vi "New Signal DVR.vi"(8 "error in (no error)":errorcluster, 11 "Signal in":refnum<class "Signal.lvclass">) -> (0 "error out":errorcluster, 3 "Signal DVR out":refnum<data-value>)   [LabVIEW 2015, in "MDSplus.lvlib" / "Signal.lvclass"]
uses:
  <vilib>/MDSplus/Classes/Data_Class/Compound_Class/Signal_Class/Signal.lvclass
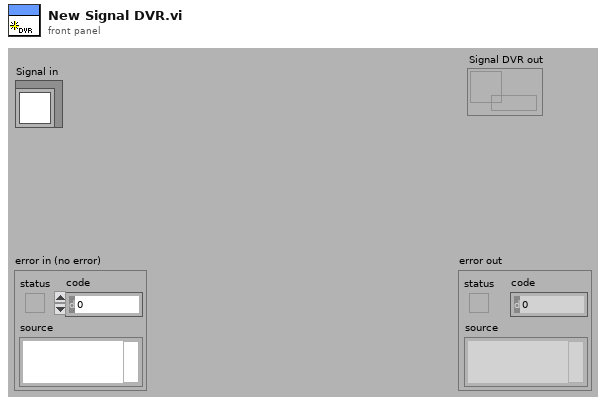
[diagram p1: front panel]
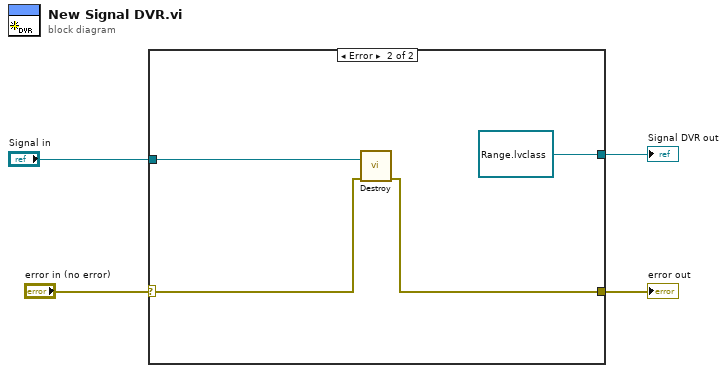
[diagram p0: block diagram]
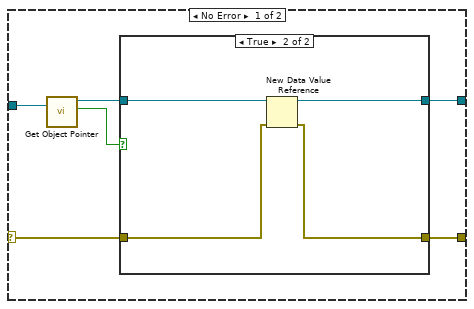
[diagram p2: hidden frame]
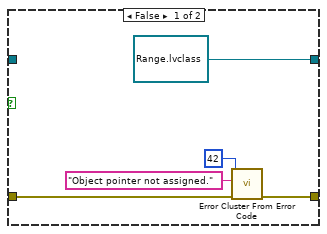
[diagram p3: hidden frame]
diagram:
  n1 = case shown="Error" "error in (no error)" {
    selector: "error in (no error)" -> [w6 w23]
    tunnel: [w10 w22] -> w4
    tunnel: [w9 refnum<data-value> refnum ("data value reference")] -> w3
    tunnel: "Signal in" -> [w5 w20]
    frame No Error {
      n2 = call-dynamic "Get Object Pointer.vi"("Data in"=w5) -> ("Assigned object pointer?"=w7:bool, "Data out"=w8:refnum<class "Signal.lvclass">)  [unwired: 8 in, 1 out]
      n3 = case shown="True" w7 {
        tunnel: w6 -> [w12 w19]
        tunnel: [w11 w16] -> w10
        tunnel: w8 -> [_ w18]
        tunnel: [refnum<data-value> refnum ("data value reference") w17] -> w9
        frame False {
          n4 = call <vilib>:"Error Cluster From Error Code.vi"("error in (no error)"=w12, "error message (\"\")"="Object pointer not assigned." ("error message (\"\")"), "error code (0)"=42) -> ("error out"=w11:errorcluster)  [unwired: 6 in]
        }
        frame True {
          n5 = New Data Value Reference(data value=w18, error in=w19) -> (data value reference=w17:refnum<data-value>, error out=w16:errorcluster)
        }
      }
    }
    frame Error {
      n6 = call-dynamic "Destroy.vi"("error in (no error)"=w23, "Signal in"=w20) -> ("error out"=w22:errorcluster)  [unwired: 9 in]
    }
  }
  "error out" <- w4
  "Signal DVR out" <- w3
